vi "Set Or get ActiveCell Bk Color.vi"(6 "Active Cell":T1 caption="活动单元格:活动单元格", 8 "error in (no error)":errorcluster caption="错误输入（无错误）", 9 "Mode":T2, 10 "BK Color In":u32(colorbox), 11 "Table Ref In":refnum<vi>) -> (0 "error out":errorcluster caption="错误输出", 2 "BK Color Out":u32(colorbox), 3 "Table Ref Out":refnum<vi>)   [LabVIEW 2013, in "Table Tool.lvlib"]
uses:
  Table Tool.lvlib
  Custum Type/GetOrSet.ctl
  <vilib>/Utility/miscctls.llb/LVRowAndColumnTypeDef.ctl
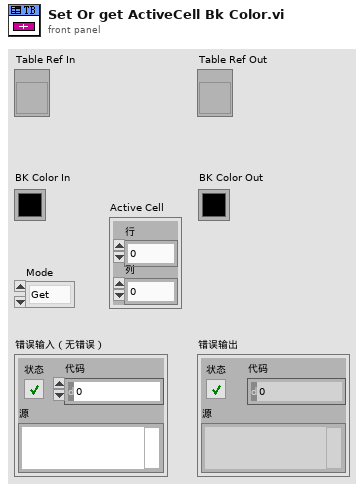
[diagram p1: front panel]
types:
  T1 = typedef "LVRowAndColumnTypeDef.ctl" = cluster{"Row":i32, "Column":i32}
  T2 = typedef "Table Tool.lvlib/GetOrSet.ctl" = enum16{"Get", "Set"}
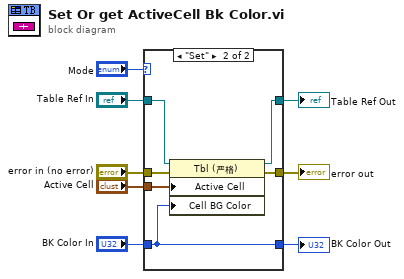
[diagram p0: block diagram]
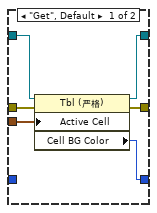
[diagram p2: hidden frame]
diagram:
  n1 = case shown="\"Set\"" "Mode" {
    tunnel: "Table Ref In" -> [w14 w19]
    tunnel: "error in (no error)" -> [w13 w20]
    tunnel: [w12 w17] -> w5
    tunnel: [w11 w18] -> w4
    tunnel: [w10 w15] -> w2
    tunnel: "BK Color In" -> [_ w15]
    tunnel: "Active Cell" -> [w9 w16]
    frame "Get", Default {
      n2 = property class="Tbl (严格)"(reference=w14, error in=w13, "Active Cell"=w9) -> (reference out=w11:refnum<vi>, error out=w12:errorcluster, "Cell BG Color"=w10:u32)
    }
    frame "Set" {
      n3 = property class="Tbl (严格)"(reference=w19, error in=w20, "Active Cell"=w16, "Cell BG Color"=w15) -> (reference out=w18:refnum<vi>, error out=w17:errorcluster)
    }
  }
  "Table Ref Out" <- w4
  "error out" <- w5
  "BK Color Out" <- w2
